vi "Display Data (SubVI).vi"(11 "Ref":refnum<vi>) -> (1 "AI Dat":dbl[](array[numeric]), 2 "DI Dat":bool[](array[boolean]), 3 "Ser Dat":string[][](array[string]))   [LabVIEW 2022 SP3]
panel:
  out "error out 7":errorcluster
  out "error out 4":errorcluster
  out "error out 2":errorcluster
  out "error out 5":errorcluster
  out "error out 6":errorcluster
  out "Array":string[](array[string])
  out "error out 3":errorcluster
  out "error out":errorcluster
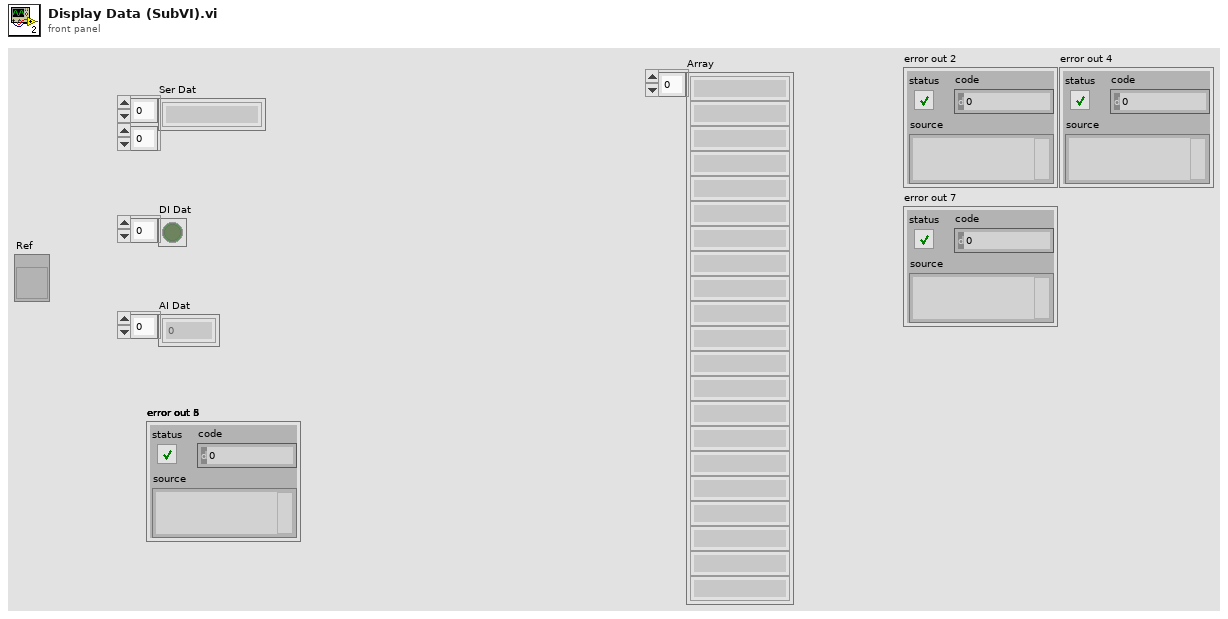
[diagram p1: front panel]
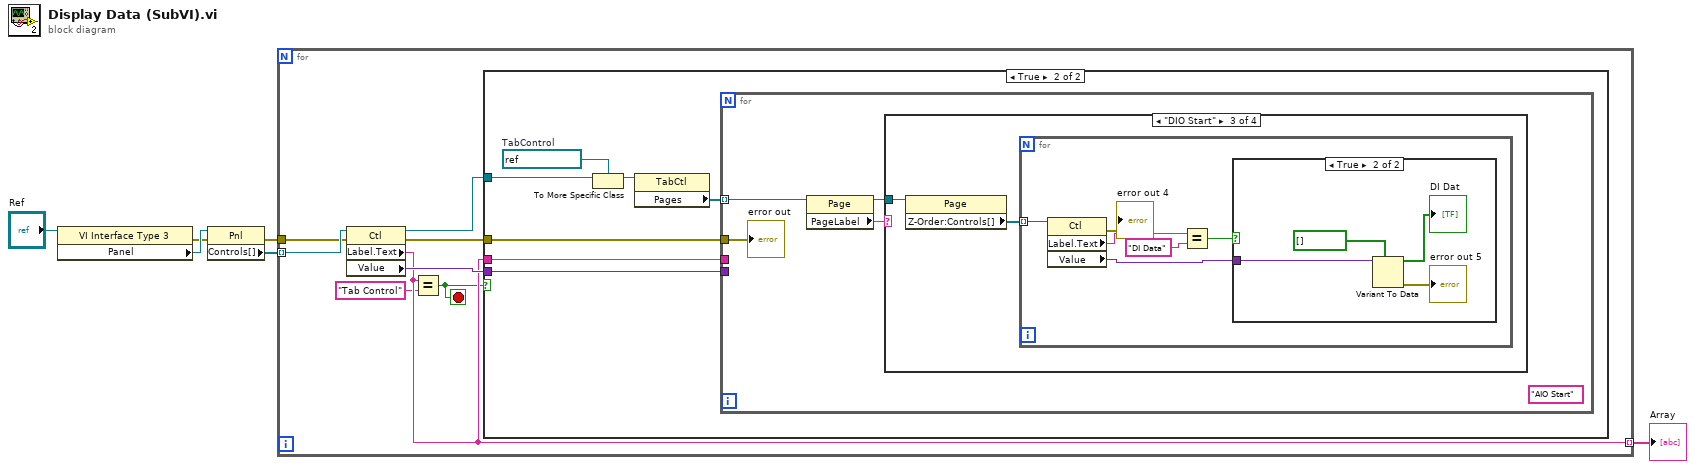
[diagram p0: block diagram]
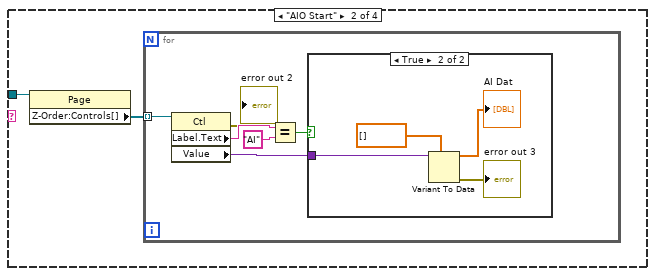
[diagram p4: hidden frame]
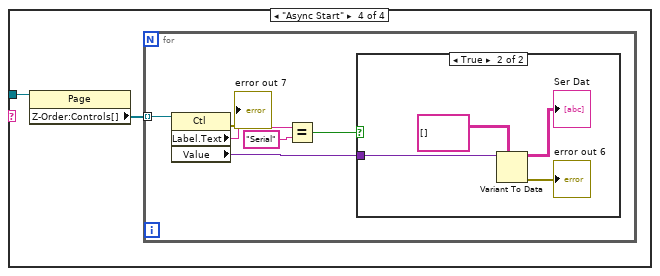
[diagram p7: hidden frame]
diagram:
  n1 = property class="VI Interface Type 3"(reference="Ref") -> (error out=w3:errorcluster, "Panel"=w6:refnum<vi>)  [unwired: 1 in, 1 out]
  n2 = property class="Pnl"(reference=w6, error in=w3) -> (error out=w2:errorcluster, "Controls[]"=w5:refnum<vi>[])  [unwired: 1 out]
  n3 = for {
    tunnel: w5 -> [w14] mode=indexing
    tunnel: w2 -> [w11]
    tunnel: [w10] -> w1 mode=indexing
    stop <- w8 stop-if-true
    n4 = property class="Ctl"(reference=w14, error in=w11) -> (reference out=w7:refnum<vi>, error out=w12:errorcluster, "Label.Text"=w10:string, "Value"=w13:variant)
    n5 = Equal?(x=w10, y="Tab Control") -> (x = y?=w8:bool)
    n6 = case shown="True" w8 {
      tunnel: w13 -> [_ w21]
      tunnel: w12 -> [_ w20]
      tunnel: w10 -> [_ w19]
      tunnel: w7 -> [_ w18]
      frame False {
      }
      frame True {
        w17 = refnum<vi> refnum  # TabControl
        n7 = To More Specific Class(target class=w17, reference=w18) -> (specific class reference=w16:refnum<vi>)  [unwired: 1 in, 1 out]
        n8 = property class="TabCtl"(reference=w16) -> ("Pages"=w15:refnum<vi>[])  [unwired: 1 in, 2 out]
        n9 = for {
          tunnel: w21 -> [_]
          tunnel: w20 -> [w25]
          tunnel: w19 -> [_]
          tunnel: w15 -> [w24] mode=indexing
          (unwired) "AIO Start" ("Label.Text")
          n10 = property class="Page"(reference=w24) -> (reference out=w22:refnum<vi>, "PageLabel"=w23:string)  [unwired: 1 in, 1 out]
          n11 = case shown="\"DIO Start\"" w23 {
            tunnel: w22 -> [_ w27 w39 w51]
            frame Default {
            }
            frame "AIO Start" {
              n12 = property class="Page"(reference=w27) -> ("Z-Order:Controls[]"=w26:refnum<vi>[])  [unwired: 1 in, 2 out]
              n13 = for {
                tunnel: w26 -> [w31] mode=indexing
                n14 = property class="Ctl"(reference=w31) -> (error out=→"error out 2":errorcluster, "Label.Text"=w30:string, "Value"=w29:variant)  [unwired: 1 in, 1 out]
                n15 = Equal?(x=w30, y="AI") -> (x = y?=w33:bool)
                n16 = case shown="True" w33 {
                  tunnel: w29 -> [_ w36]
                  frame False {
                  }
                  frame True {
                    n17 = Variant To Data(type=dbl[] [], Variant=w36) -> (data=→"AI Dat":dbl[], error out=→"error out 3":errorcluster)  [unwired: 1 in]
                  }
                }
              }
            }
            frame "DIO Start" {
              n18 = property class="Page"(reference=w39) -> ("Z-Order:Controls[]"=w38:refnum<vi>[])  [unwired: 1 in, 2 out]
              n19 = for {
                tunnel: w38 -> [w43] mode=indexing
                n20 = property class="Ctl"(reference=w43) -> (error out=→"error out 4":errorcluster, "Label.Text"=w42:string, "Value"=w41:variant)  [unwired: 1 in, 1 out]
                n21 = Equal?(x=w42, y="DI Data") -> (x = y?=w45:bool)
                n22 = case shown="True" w45 {
                  tunnel: w41 -> [_ w49]
                  frame False {
                  }
                  frame True {
                    n23 = Variant To Data(type=bool[] [], Variant=w49) -> (data=→"DI Dat":bool[], error out=→"error out 5":errorcluster)  [unwired: 1 in]
                  }
                }
              }
            }
            frame "Async Start" {
              n24 = property class="Page"(reference=w51) -> ("Z-Order:Controls[]"=w50:refnum<vi>[])  [unwired: 1 in, 2 out]
              n25 = for {
                tunnel: w50 -> [w55] mode=indexing
                n26 = property class="Ctl"(reference=w55) -> (error out=→"error out 7":errorcluster, "Label.Text"=w54:string, "Value"=w53:variant)  [unwired: 1 in, 1 out]
                n27 = Equal?(x=w54, y="Serial") -> (x = y?=w57:bool)
                n28 = case shown="True" w57 {
                  tunnel: w53 -> [_ w60]
                  frame False {
                  }
                  frame True {
                    n29 = Variant To Data(type=string[][] [], Variant=w60) -> (data=→"Ser Dat":string[][], error out=→"error out 6":errorcluster)  [unwired: 1 in]
                  }
                }
              }
            }
          }
          "error out" <- w25
        }
      }
    }
  }
  "Array" <- w1
